vi "Convert TreeTestTag into Execution Tag Hierarchy.vi"(8 "error in":errorcluster, 10 "TestTag":string, 11 "Tree reference":refnum<vi>) -> (0 "error out":errorcluster, 2 "Test Tags to Execute":string[](array[string]))   [LabVIEW 2011, in "GraphicalTestRunner.lvlib"]
uses:
  GraphicalTestRunner.lvlib
  JKI Reuse/Filter Error Codes (Scalar)__jki_lib_error_handling -- VI Tester.vi
  <userlib>/_OpenG.lib/array/array.llb/Remove Duplicates from 1D Array (String)__ogtk.vi
  <userlib>/_OpenG.lib/array/array.llb/Filter 1D Array (String)__ogtk.vi
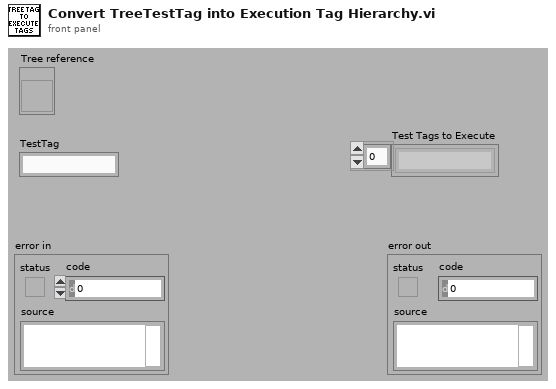
[diagram p1: front panel]
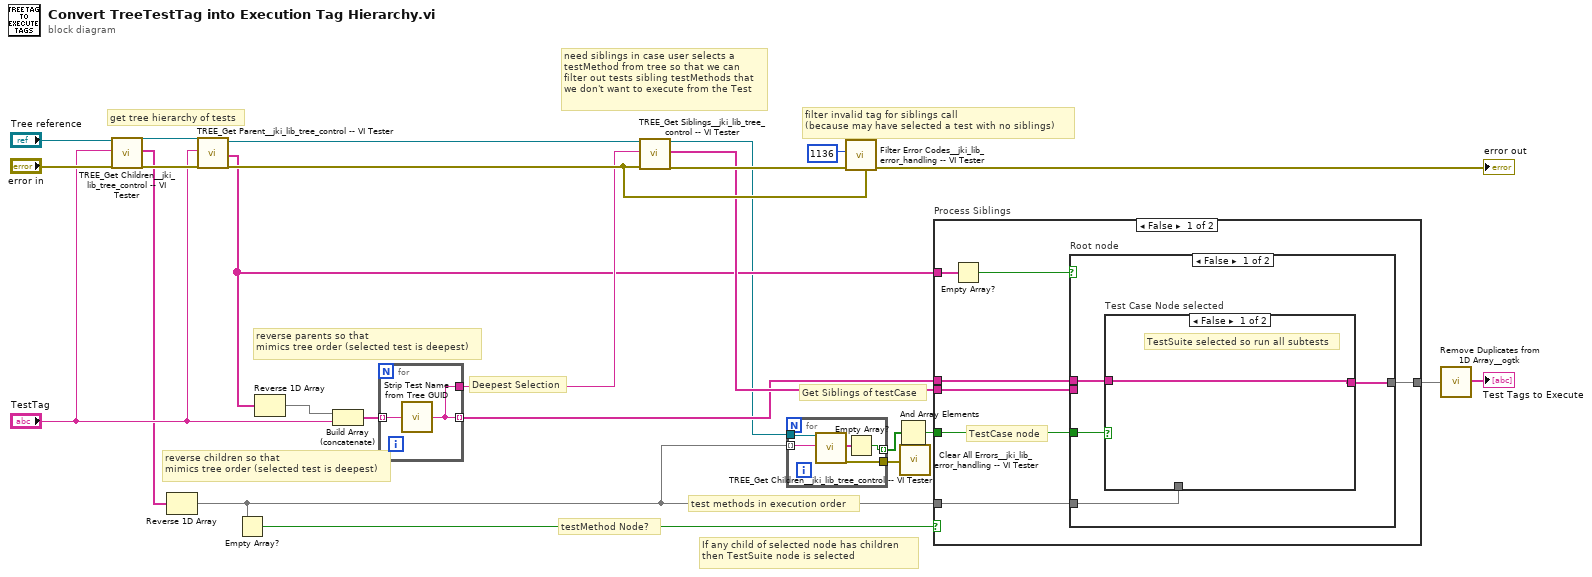
[diagram p0: block diagram]
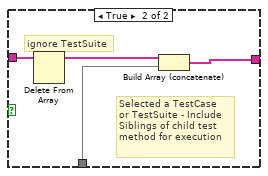
[diagram p2: hidden frame]
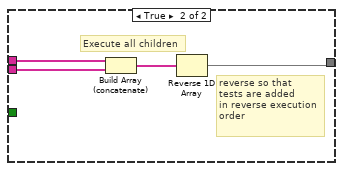
[diagram p3: hidden frame]
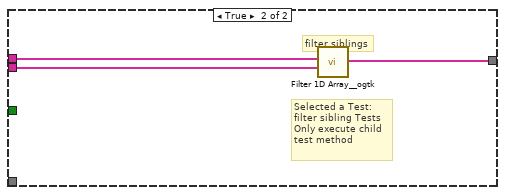
[diagram p4: hidden frame]
diagram:
  # "If any child of selected node has children\nthen TestSuite node is selected"
  # "need siblings in case user selects a testMethod from tree so that we can filter out tests sibling testMethods that we don't want to execute from the Test"
  # "reverse children so that\nmimics tree order (selected test is deepest)"
  # "test methods in execution order"
  # "Deepest Selection"
  # "Get Siblings of testCase"
  # "reverse parents so that\nmimics tree order (selected test is deepest)"
  # "get tree hierarchy of tests"
  # "filter invalid tag for siblings call\n(because may have selected a test with no siblings)"
  # "testMethod Node?"
  n1 = call "TREE_Get Children__jki_lib_tree_control -- VI Tester.vi"("Tree Reference In"="Tree reference", "Parent Tag"="TestTag", "error in (no error)"="error in") -> ("Tree Reference Out"=w13:refnum<vi>, "Children Tags"=w7:string[], "error out"=w20:errorcluster)  [unwired: 14 in]
  n2 = Reverse 1D Array(array=w7) -> (reversed array=w4:string[])
  n3 = call "TREE_Get Parent__jki_lib_tree_control -- VI Tester.vi"("Tree Reference In"=w13, "Child Tag (Current)"="TestTag", "error in (no error)"=w20) -> ("Tree Reference Out"=w15:refnum<vi>, "Parents Tags"=w6:string[], "error out"=w23:errorcluster)  [unwired: 13 in, 1 out]
  n4 = Empty Array?(array=w4) -> (empty?=w8:bool)
  n5 = Reverse 1D Array(array=w6) -> (reversed array=w14:string[])
  n6 = Build Array (concatenate)(w14, "TestTag") -> (w17:string[])
  n7 = for {
    tunnel: w17 -> [w27] mode=indexing
    tunnel: [w26] -> w10 mode=indexing
    tunnel: [w26] -> w19
    n8 = call "Strip Test Name from Tree GUID.vi"("TestTag GUID"=w27) -> ("Test GUID"=w26:string)
  }
  n9 = call "TREE_Get Siblings__jki_lib_tree_control -- VI Tester.vi"("Tree Reference In"=w15, "Input Tag (Current)"=w19, "error in (no error)"=w23) -> ("Tree Reference Out"=w5:refnum<vi>, "Sibling Tags"=w16:string[], "error out"=w21:errorcluster)  [unwired: 14 in]
  n10 = for {
    tunnel: w5 -> [w32]
    tunnel: w4 -> [w30] mode=indexing
    tunnel: [w31] -> w3
    tunnel: [w28] -> w2 mode=indexing
    n11 = call "TREE_Get Children__jki_lib_tree_control -- VI Tester.vi"("Tree Reference In"=w32, "Parent Tag"=w30) -> ("Children Tags"=w29:string[], "error out"=w31:errorcluster)  [unwired: 15 in, 1 out]
    n12 = Empty Array?(array=w29) -> (empty?=w28:bool)
  }
  n13 = call-poly "Filter Error Codes__jki_lib_error_handling -- VI Tester.vi"("upstream error (optional)"=w23, "error in"=w21, "error code to filter"=1136) -> ("error out"=→"error out":errorcluster)  [unwired: 6 in, 2 out]
  n14 = And Array Elements(Boolean array=w2) -> (logical AND=w1:bool)
  n15 = call "Clear All Errors__jki_lib_error_handling -- VI Tester.vi"("error in"=w3) -> ()  [unwired: 4 in, 1 out]
  n16 = case "Process Siblings" shown="False" w8 {
    tunnel: w16 -> [w34 w55]
    tunnel: w10 -> [w38 w54]
    tunnel: [w39 w53] -> w18
    tunnel: w4 -> [w37 _]
    tunnel: w6 -> [w36 _]
    tunnel: w1 -> [w33 _]
    frame False {
      # "TestCase node"
      n17 = Empty Array?(array=w36) -> (empty?=w35:bool)
      n18 = case "Root node" shown="False" w35 {
        tunnel: [w43 w50] -> w39
        tunnel: w38 -> [w42 w52]
        tunnel: w37 -> [w41 _]
        tunnel: w34 -> [_ w51]
        tunnel: w33 -> [w40 _]
        frame False {
          n19 = case "Test Case Node selected" shown="False" w40 {
            tunnel: [w44 w48] -> w43
            tunnel: w42 -> [w44 w47]
            tunnel: w41 -> [_ w45]
            frame False {
              # "TestSuite selected so run all subtests"
            }
            frame True {
              # "ignore TestSuite"
              # "Selected a TestCase\nor TestSuite - Include\nSiblings of child test\nmethod for execution"
              n20 = Delete From Array(array=w47) -> (array with subset deleted=w46:string[])  [unwired: 2 in, 1 out]
              n21 = Build Array (concatenate)(w46, w45) -> (w48:string[])
            }
          }
        }
        frame True {
          # "reverse so that\ntests are added\nin reverse execution\norder"
          # "Execute all children"
          n22 = Build Array (concatenate)(w52, w51) -> (w49:string[])
          n23 = Reverse 1D Array(array=w49) -> (reversed array=w50:string[])
        }
      }
    }
    frame True {
      # "filter siblings"
      # "Selected a Test:\nfilter sibling Tests\nOnly execute child\ntest method"
      n24 = call-poly <userlib>:"Filter 1D Array__ogtk.vi"("items to filter"=w55, "array"=w54) -> ("filtered array"=w53:string[])  [unwired: 4 in, 1 out]
    }
  }
  n25 = call-poly <userlib>:"Remove Duplicates from 1D Array__ogtk.vi"("Input Array"=w18) -> ("Output Array"=→"Test Tags to Execute":string[])  [unwired: 1 out]
